vi "Reset.vi"(8 "error in (no error)":errorcluster, 11 "GEN40-38-LAN in":refnum<class "GEN40-38-LAN.lvclass">) -> (0 "error out":errorcluster, 3 "GEN40-38-LAN out":refnum<class "GEN40-38-LAN.lvclass">)   [LabVIEW 2018, in "GEN40-38-LAN.lvlib" / "GEN40-38-LAN.lvclass"]
uses:
  GEN40-38-LAN.lvclass
  PPLs/Power Supply/Parent/Power_Supply.lvlibp/Power Supply.lvclass
  C:/Projects/LabVIEW/PPLs/Power Supply/Parent/Power_Supply.lvlibp/Power Supply.lvclass
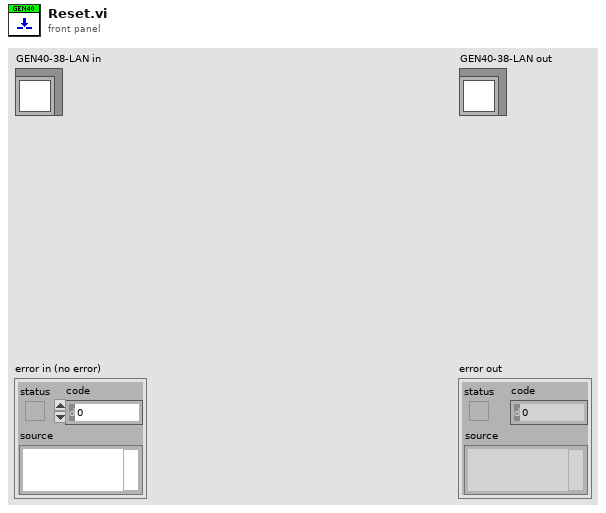
[diagram p1: front panel]
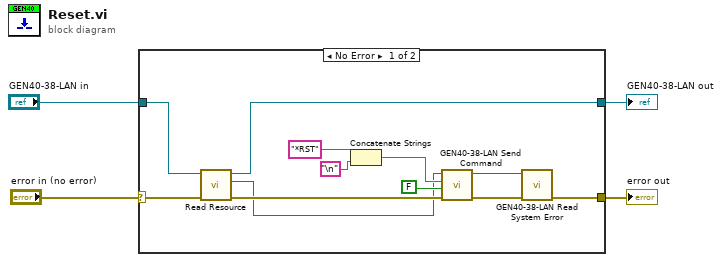
[diagram p0: block diagram]
diagram:
  n1 = case shown="No Error" "error in (no error)" {
    selector: "error in (no error)" -> [w16 w18]
    tunnel: [w5 w18] -> w3
    tunnel: [w8 w17] -> w2
    tunnel: "GEN40-38-LAN in" -> [w15 w17]
    frame No Error {
      n2 = call "Read Resource.vi"("error in"=w16, "Power Supply in"=w15) -> ("error out"=w11:errorcluster, "Resource"=w10:refnum<visa-resource-name>, "Power Supply out"=w8:refnum<class "GEN40-38-LAN.lvclass">)  [unwired: 7 in]
      n3 = Concatenate Strings("*RST" ("string"), "\n" ("string")) -> (w13:string)
      n4 = call "GEN40-38-LAN Send Command.vi"("error in (no error)"=w11, "Wait for Response?"=FALSE, "Command"=w13, "VISA resource name"=w10) -> ("error out"=w6:errorcluster, "VISA resource name out"=w7:refnum<visa-resource-name>)  [unwired: 5 in, 1 out]
      n5 = call "GEN40-38-LAN Read System Error.vi"("error in (no error)"=w6, "Resource"=w7) -> ("error out"=w5:errorcluster)  [unwired: 9 in]
    }
    frame Error {
    }
  }
  "error out" <- w3
  "GEN40-38-LAN out" <- w2
